vi "Convert State For Save.vi"(2 "Container State":T1, 3 "Display State":T2) -> (1 "Display State To Save":variant)   [LabVIEW 2020, in "MGI Path Selector.xctl"]
uses:
  <userlib>/_MGI/User Interface/Path Selector XControl/MGI Path Selector.xctl
  <userlib>/_MGI/User Interface/Path Selector XControl/State.ctl
  <userlib>/_MGI/User Interface/Path Selector XControl/Class Hierarchy/MGI Path Selector.lvclass
  <vilib>/_xctls/Container State.ctl
  <vilib>/_xctls/XControlSupport.lvlib
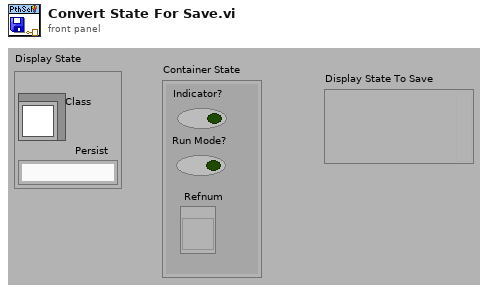
[diagram p1: front panel]
types:
  T1 = typedef "XControlSupport.lvlib/Container State.ctl" = cluster{"Indicator?":bool, "Run Mode?":bool, " Refnum":refnum<vi>}
  T2 = typedef "MGI Path Selector.xctl/State.ctl" = cluster{"Class":refnum<class "MGI Path Selector.lvclass">, "Persist":string}
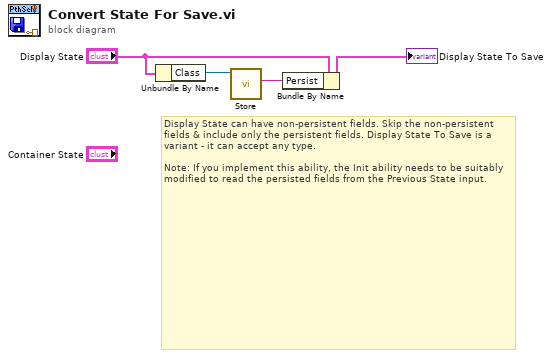
[diagram p0: block diagram]
diagram:
  # "Display State can have non-persistent fields. Skip the non-persistent fields & include only the persistent fields. Display State To Save is a variant - it can accept any type.\n\nNote: If you implement this ability, the Init ability needs to be suitably modified to read the persisted fields from the Previous State input."
  n1 = Unbundle By Name("Display State") -> ("Class"=w4:refnum<class "MGI Path Selector.lvclass">)
  n2 = call-dynamic "Store.vi"("Path Selector in"=w4) -> ("String"=w3:string)  [unwired: 9 in, 1 out]
  n3 = Bundle By Name(cluster="Display State", "Persist"=w3) -> (→"Display State To Save":T2)
